vi "setUp.vi"(8 "error in (no error)":errorcluster, 11 "reference in":refnum<class "VI Tester Setup Error.lvclass">) -> (0 "error out":errorcluster, 3 "reference out":refnum<class "VI Tester Setup Error.lvclass">)   [LabVIEW 2020, in "VI Tester Setup Error.lvclass"]
doc: "setUp runs prior to the test method during test execution. Use this method to initialize any object data required by your tests."
uses:
  VI Tester Setup Error.lvclass
  C:/Program Files (x86)/National Instruments/LabVIEW 2020/vi.lib/addons/_JKI Toolkits/VI Tester/TestCase.llb/TestCase.lvclass
  VI Tester Setup Error.lvclass/VI Tester Setup Error.ctl
  <vilib>/addons/_JKI Toolkits/VI Tester/TestCase.llb/TestCase.lvclass
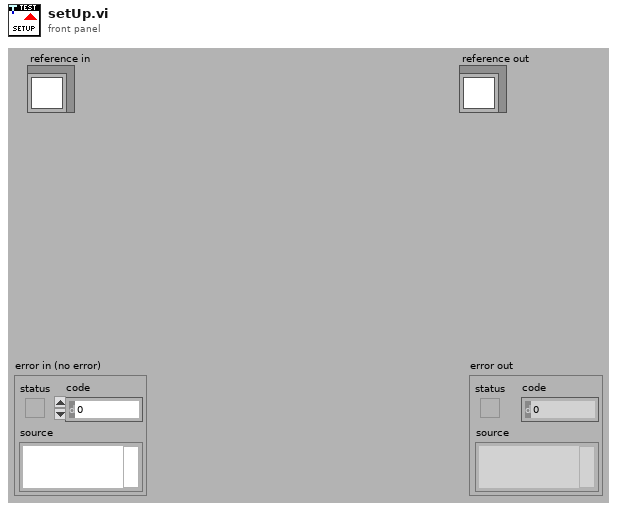
[diagram p1: front panel]
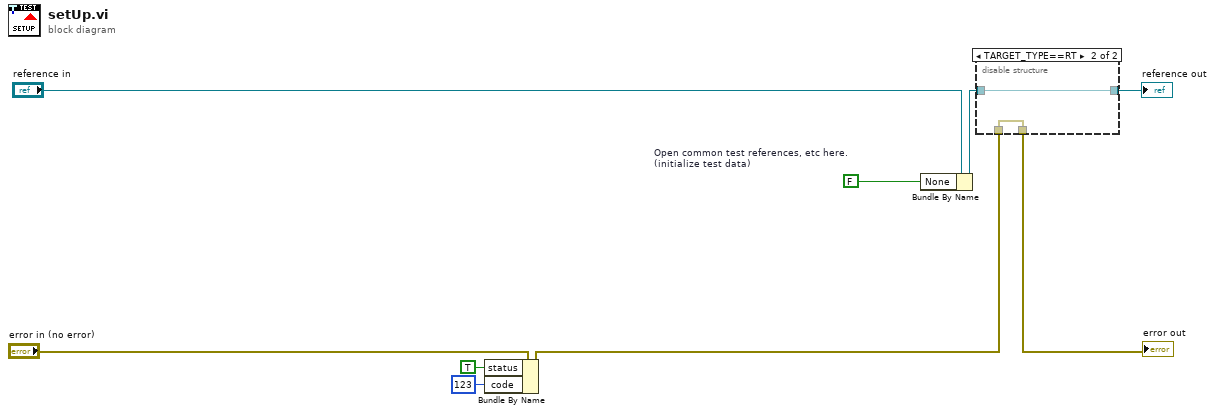
[diagram p0: block diagram]
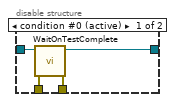
[diagram p2: hidden frame]
diagram:
  w4 = FALSE  # Open common test references, etc here. (initialize test data)
  n1 = Bundle By Name(cluster="error in (no error)", "status"=TRUE, "code"=123) -> (w3:errorcluster)
  n2 = Bundle By Name(cluster="reference in", "None"=w4) -> (w5:refnum<class "VI Tester Setup Error.lvclass">)
  n3 = disable-structure shown="TARGET_TYPE==RT" {
    disable-tunnel: w3 -> [w13 w14]
    disable-tunnel: [w12 w14] -> w8
    disable-tunnel: [w11 w15] -> w6
    disable-tunnel: w5 -> [w10 w15]
    frame condition #0 (active) {
      n4 = call <vilib>:"WaitOnTestComplete.vi"("error in (no error)"=w13, "TestCase in"=w10) -> ("error out"=w12:errorcluster, "TestCase out"=w11:refnum<class "VI Tester Setup Error.lvclass">)  [unwired: 8 in]
    }
    frame condition #1 {
    }
  }
  "error out" <- w8
  "reference out" <- w6
